vi "Wrap Data for Measurement Logic Initialization.vi"(11 "measurement configuration":T5={"config"="SI1", "BITFILE"=""}) -> (0 "REF. CLOCK  (Hz)":dbl, 1 "RIO HANDLER":string, 2 "CSI-2 DATA SOURCE":u32, 3 "Serial Input Configuration":T6[](array[typedef]) {"RAW Display Parameters"."Bayer Parameters"."Blue Gain" min=0.0 max=3.99 step=0.1 format="%_4g"; "RAW Display Parameters"."Bayer Parameters"."Green Gain" min=0.0 max=3.99 step=0.1 format="%_4g"; "RAW Display Parameters"."Bayer Parameters"."Red Gain" min=0.0 max=3.99 step=0.1 format="%_4g"; "RAW Display Parameters"."Bayer Parameters"."Algorithm" items=["Bilinear", "VNG"]; "RAW Display Parameters"."Bayer Parameters"."Pattern" items=["GB", "GR", "BG", "RG"]}, 4 "POC SOURCE":u32, 5 "appended path":path, 6 "SI ACTIVE LANE CNT":u32, 7 "PATH TO CONFIGURATION SCRIPT":string, 8 "config":T1)   [LabVIEW 2025, in "Automotive Vision.lvclass"]
doc: "Wraps data for the logic initialization, convert data from the measurement configuration to the logic."
uses:
  Automotive Vision.lvclass
  Automotive Vision.lvclass/Automotive Vision.ctl
  <instrlib>/FlexRIO/CSI-2/v2/Common/Types/LLP Data Type.ctl
  <instrlib>/FlexRIO/CSI-2/v2/Common/NI CSI-2 API Common v2.lvlib
  <instrlib>/FlexRIO/CSI-2/v2/FPGA/Types/Display Parameters.ctl
  <instrlib>/FlexRIO/CSI-2/v2/FPGA/NI CSI-2 API FPGA v2.lvlib
  ttashjia/GSE/Host/Common/Types/RAW Interpretation for Display.ctl
  ttashjia/GSE/Host/Common/GettingStarted_Common_148X_Host.lvlib
  ttashjia/GSE/Host/Common/Types/Serial Channel Configuration.ctl
  embedded data item.ctl
  embedded data.ctl
  autovision_config.ctl
  register.ctl
  Measurement Configuration.ctl
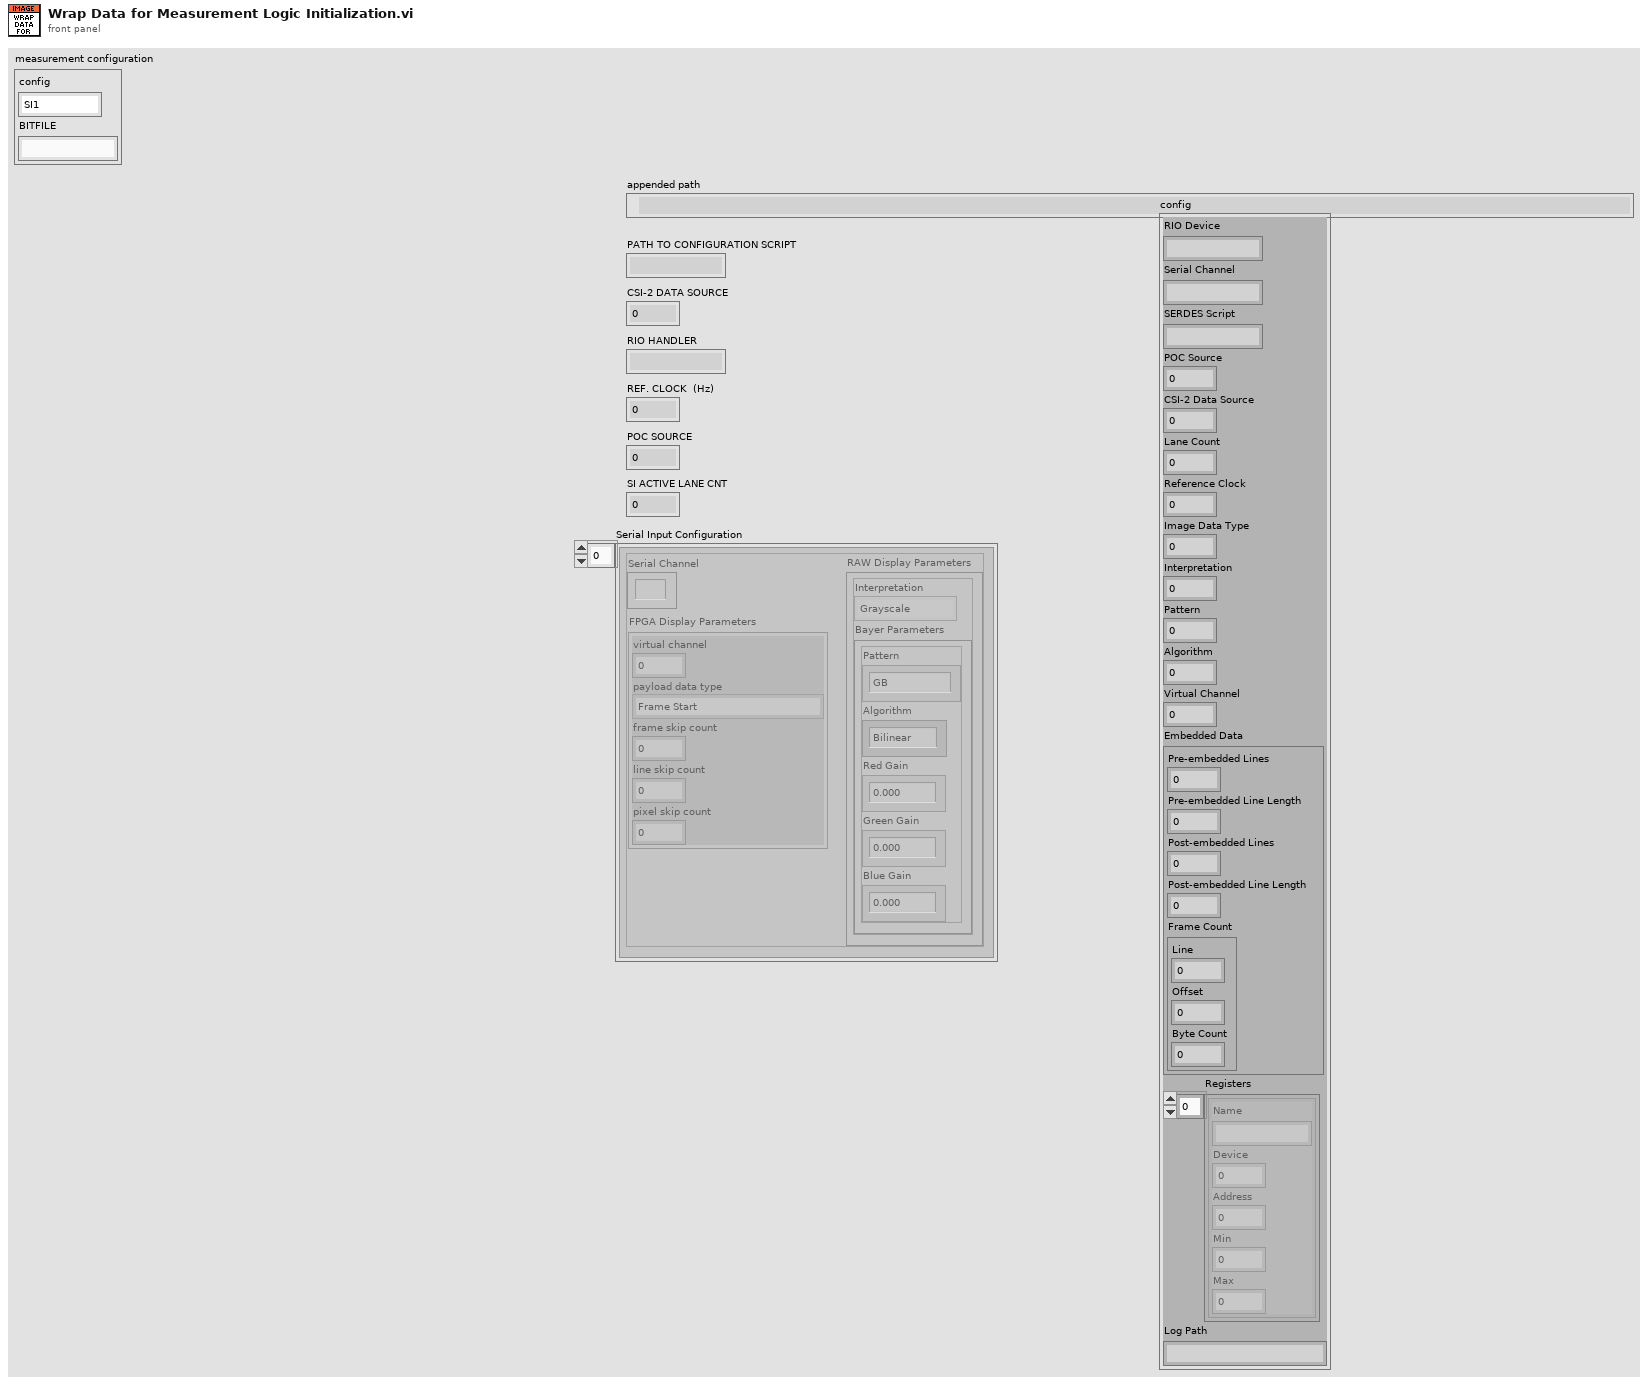
[diagram p1: front panel]
types:
  T1 = typedef "Automotive Vision.lvclass/autovision_config.ctl" = cluster{"RIO Device":string, "Serial Channel":string, "SERDES Script":string, "POC Source":u32, "CSI-2 Data Source":u32, "Lane Count":u32, "Reference Clock":dbl, "Image Data Type":u32, "Interpretation":u32, "Pattern":u32, "Algorithm":u32, "Virtual Channel":u32, "Embedded Data":T2, "Registers":T4[], "Log Path":string}
  T2 = typedef "Automotive Vision.lvclass/embedded data.ctl" = cluster{"Pre-embedded Lines":dbl, "Pre-embedded Line Length":dbl, "Post-embedded Lines":dbl, "Post-embedded Line Length":dbl, "Frame Count":T3}
  T3 = typedef "Automotive Vision.lvclass/embedded data item.ctl" = cluster{"Line":dbl, "Offset":dbl, "Byte Count":dbl}
  T4 = typedef "Automotive Vision.lvclass/register.ctl" = cluster{"Name":string, "Device":u8, "Address":u16, "Min":u16, "Max":u16}
  T5 = typedef "Automotive Vision.lvclass/Measurement Configuration.ctl" = cluster{"config":string, "BITFILE":string}
  T6 = typedef "GettingStarted_Common_148X_Host.lvlib/Serial Channel Configuration.ctl" = cluster{"Serial Channel":string, "FPGA Display Parameters":T7, "RAW Display Parameters":cluster{"Interpretation":T9, "Bayer Parameters":cluster{"Pattern":i32, "Algorithm":i32, "Red Gain":dbl, "Green Gain":dbl, "Blue Gain":dbl}}}
  T7 = typedef "NI CSI-2 API FPGA v2.lvlib/Display Parameters.ctl" = cluster{"virtual channel":fxp<+,4,4>, "payload data type":T8, "frame skip count":u16, "line skip count":u8, "pixel skip count":fxp<+,5,5>}
  T8 = typedef "NI CSI-2 API Common v2.lvlib/LLP Data Type.ctl" = enum8{"Frame Start", "Frame End", "Line Start", "Line End", "End of Transmission", "Reserved 0", "Reserved 1", "Reserved 2", "Generic Short Packet 1", "Generic Short Packet 2", "Generic Short Packet 3", "Generic Short Packet 4", "Generic Short Packet 5", "Generic Short Packet 6", "Generic Short Packet 7", "Generic Short Packet 8", "Null", "Blanking Data", "Embedded 8-bit non Image Data", "Generic Long Packet 1", "Generic Long Packet 2", "Generic Long Packet 3", "Generic Long Packet 4", "Reserved 3", "YUV420 8-bit", "YUV420 10-bit", "Legacy YUV420 8-bit", "Reserved 4", "YUV420 8-bit Chroma Shifted", "YUV420 10-bit Chroma Shifted", "YUV422 8-bit", "YUV422 10-bit", "RGB444", "RGB555", "RGB565", "RGB666", "RGB888", "Reserved 5", "Reserved 6", "RAW 24", "RAW 6", "RAW 7", "RAW 8", "RAW 10", "RAW 12", "RAW 14", "RAW 16", "RAW 20", "User Defined 8-bit Data 1", "User Defined 8-bit Data 2", "User Defined 8-bit Data 3", "User Defined 8-bit Data 4", "User Defined 8-bit Data 5", "User Defined 8-bit Data 6", "User Defined 8-bit Data 7", "User Defined 8-bit Data 8", "USL Command", "Reserved 7", "Reserved 8", "Reserved 9", "Reserved 10", "Reserved 11", "Reserved 12", "LRTE EPD Spacer"}
  T9 = typedef "GettingStarted_Common_148X_Host.lvlib/RAW Interpretation for Display.ctl" = enum16{"Grayscale", "Bayer", "RGB", "YUV422", "YUV420", "Legacy YUV420"}
  T10 = cluster{"Pattern":i32, "Algorithm":i32, "Red Gain":dbl, "Green Gain":dbl, "Blue Gain":dbl}
  T11 = cluster{"Interpretation":T9, "Bayer Parameters":cluster{"Pattern":i32, "Algorithm":i32, "Red Gain":dbl, "Green Gain":dbl, "Blue Gain":dbl}}
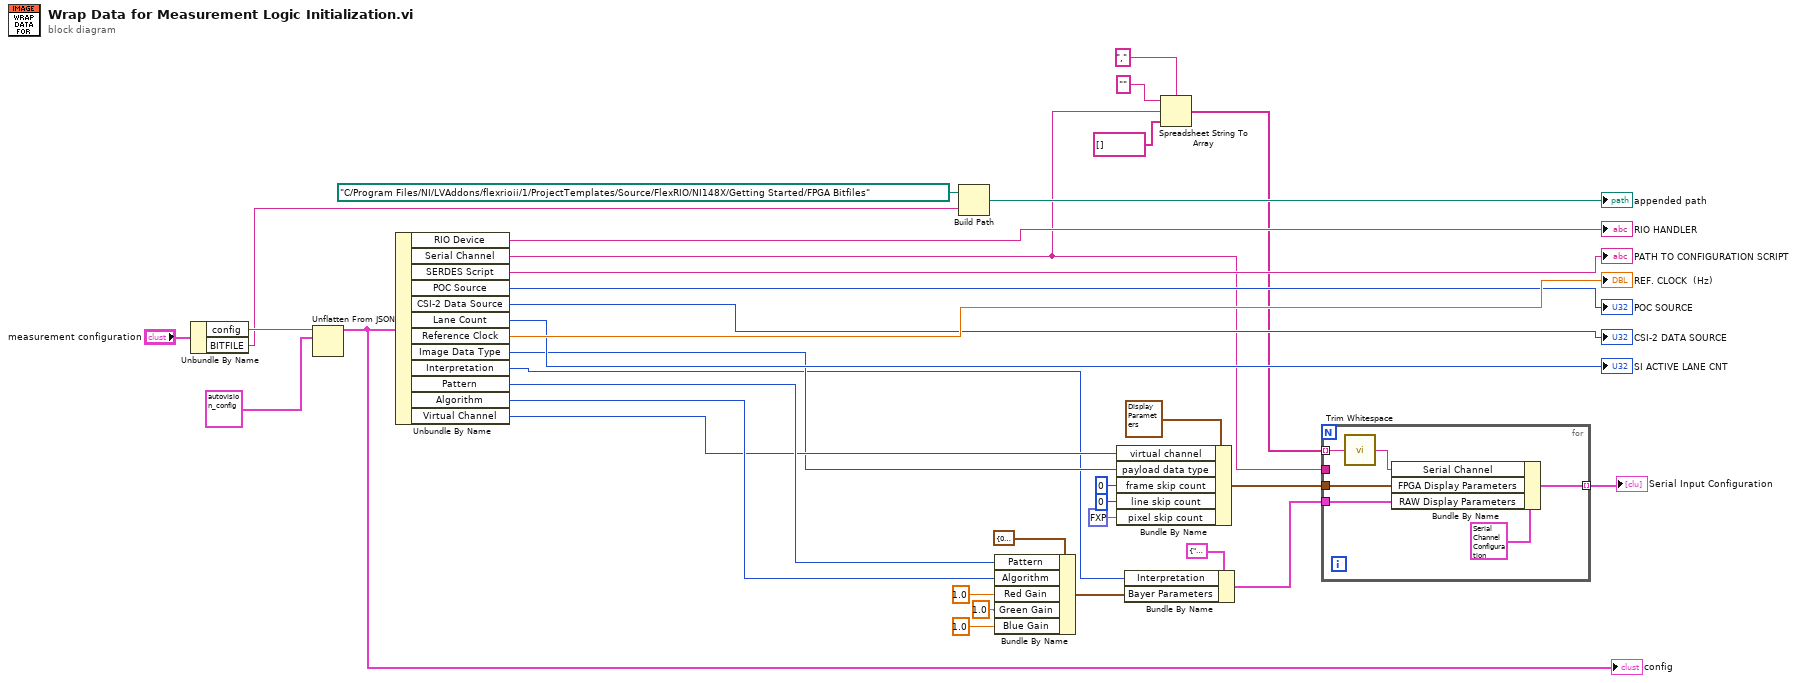
[diagram p0: block diagram]
diagram:
  n1 = Unbundle By Name("measurement configuration") -> ("config"=w9:string, "BITFILE"=w7:string)
  n2 = Unflatten From JSON(JSON string=w9, type and defaults=T1 {"RIO Device"="", "Serial Channel"="", "SERDES Script"="", "POC Source"=0, "CSI-2 Data Source"=0, "Lane Count"=0, "Reference Clock"=0.0, "Image Data Type"=0, "Interpretation"=0, "Pattern"=0, "Algorithm"=0, "Virtual Channel"=0, "Embedded Data"={"Pre-embedded Lines"=0.0, "Pre-embedded Line Length"=0.0, "Post-embedded Lines"=0.0, "Post-embedded Line Length"=0.0, "Frame Count"={"Line"=0.0, "Offset"=0.0, "Byte Count"=0.0}}, "Registers"=[], "Log Path"=""} ("Auto Vision Config")) -> (value=w8:T1)  [unwired: 5 in, 1 out]
  "config" <- w8
  n3 = Unbundle By Name(w8) -> ("RIO Device"=→"RIO HANDLER":string, "Serial Channel"=w2:string, "SERDES Script"=→"PATH TO CONFIGURATION SCRIPT":string, "POC Source"=→"POC SOURCE":u32, "CSI-2 Data Source"=→"CSI-2 DATA SOURCE":u32, "Lane Count"=→"SI ACTIVE LANE CNT":u32, "Reference Clock"=→"REF. CLOCK  (Hz)":dbl, "Image Data Type"=w12:u32, "Interpretation"=w6:u32, "Pattern"=w15:u32, "Algorithm"=w14:u32, "Virtual Channel"=w13:u32)
  n4 = Build Path(base path=path "C:/Program Files/NI/LVAddons/flexrioii/1/ProjectTemplates/Source/FlexRIO/NI148X/Getting Started/FPGA Bitfiles", name or relative path=w7) -> (appended path=→"appended path":path)
  n5 = Bundle By Name(cluster=T10 {"Pattern"=0, "Algorithm"=0, "Red Gain"=0.0, "Green Gain"=0.0, "Blue Gain"=0.0} ("Bayer Parameters"), "Pattern"=w15, "Algorithm"=w14, "Red Gain"=1.0, "Green Gain"=1.0, "Blue Gain"=1.0) -> (w30:T10)
  n6 = Bundle By Name(cluster=T7 {"virtual channel"=0.0, "payload data type"=enum."Frame Start", "frame skip count"=0, "line skip count"=0, "pixel skip count"=0.0} ("FPGA Display Parameters"), "virtual channel"=w13, "payload data type"=w12, "frame skip count"=u16 0, "line skip count"=u8 0, "pixel skip count"=fxp<+,5,5> 0.0) -> (w27:T7)
  n7 = Bundle By Name(cluster=T11 {"Interpretation"=enum."Grayscale", "Bayer Parameters"={"Pattern"=0, "Algorithm"=0, "Red Gain"=0.0, "Green Gain"=0.0, "Blue Gain"=0.0}} ("RAW Display Parameters"), "Interpretation"=w6, "Bayer Parameters"=w30) -> (w34:T11)
  n8 = Spreadsheet String To Array(delimiter (Tab)=",", format string="", spreadsheet string=w2, array type (2D Dbl)=string[] []) -> (array=w1:string[])
  n9 = for {
    tunnel: [w42] -> w35 mode=indexing
    tunnel: w34 -> [w41]
    tunnel: w27 -> [w40]
    tunnel: w2 -> [_]
    tunnel: w1 -> [w38] mode=indexing
    n10 = call <vilib>:"Trim Whitespace.vi"("string"=w38) -> ("trimmed string"=w37:string)  [unwired: 1 in]
    n11 = Bundle By Name(cluster=T6 {"Serial Channel"="SI0", "FPGA Display Parameters"={"virtual channel"=0.0, "payload data type"=enum."RAW 12", "frame skip count"=0, "line skip count"=0, "pixel skip count"=0.0}, "RAW Display Parameters"={"Interpretation"=enum."Bayer", "Bayer Parameters"={"Pattern"=3, "Algorithm"=0, "Red Gain"=1.0, "Green Gain"=1.0, "Blue Gain"=1.0}}} ("Channel Configurations element"), "Serial Channel"=w37, "FPGA Display Parameters"=w40, "RAW Display Parameters"=w41) -> (w42:T6)
  }
  "Serial Input Configuration" <- w35
